vi "LVPortMessageDataToVariant.vi"(9 "Message Data Object":variant, 10 "Value type (or value to update)":variant, 11 "pID":string) -> (3 "Value":variant)   [LabVIEW 2017]
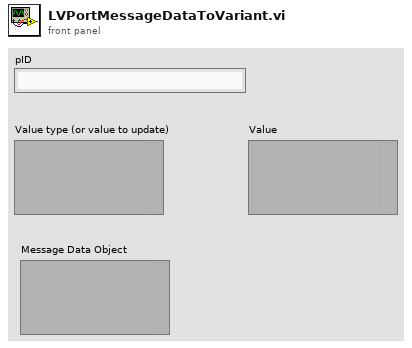
[diagram p1: front panel]
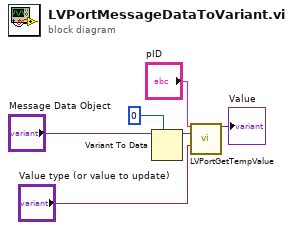
[diagram p0: block diagram]
diagram:
  n1 = Variant To Data(type=0, Variant="Message Data Object") -> (data=w3:i32)  [unwired: 1 in, 1 out]
  n2 = call "LVPortGetTempValue.vi"("pID"="pID", "Object ID"=w3, "Value Type (Or value to update)"="Value type (or value to update)") -> ("Value"=→"Value":variant)  [unwired: 10 in, 2 out]
